vi "Book rotx_pi_2.vi"() -> ()   [LabVIEW 2013]
uses:
  <vilib>/Analysis/Matrix/Datatypes/ComplexMatrix.ctl
  <vilib>/Analysis/7linalg.llb/Real Eigenvalues and Vectors.vi
  <vilib>/robotics/Kinematics/NI_Kinematics.lvlib
  <vilib>/Analysis/NI_AALPro.lvlib
  <vilib>/picture/3D Picture Control/NI_3D Picture Control.lvlib
  <vilib>/Analysis/Matrix/NI_Matrix.lvlib
panel:
  out "rot Y * rot X":picture
  out "3D Picture 3":refnum<vi>(3d-picture)
  out "rot X * rot Y":picture
  out "3D Picture 2":refnum<vi>(3d-picture)
  out "3D Picture":refnum<vi>(3d-picture)
  out "RPY transformation":picture
  out "transformation matrix":picture
  out "Eigenvectors":T1
  out "Eigenvalues":cdb[](array[numeric])
  out "vector":dbl[](array[numeric])
  out "theta":dbl
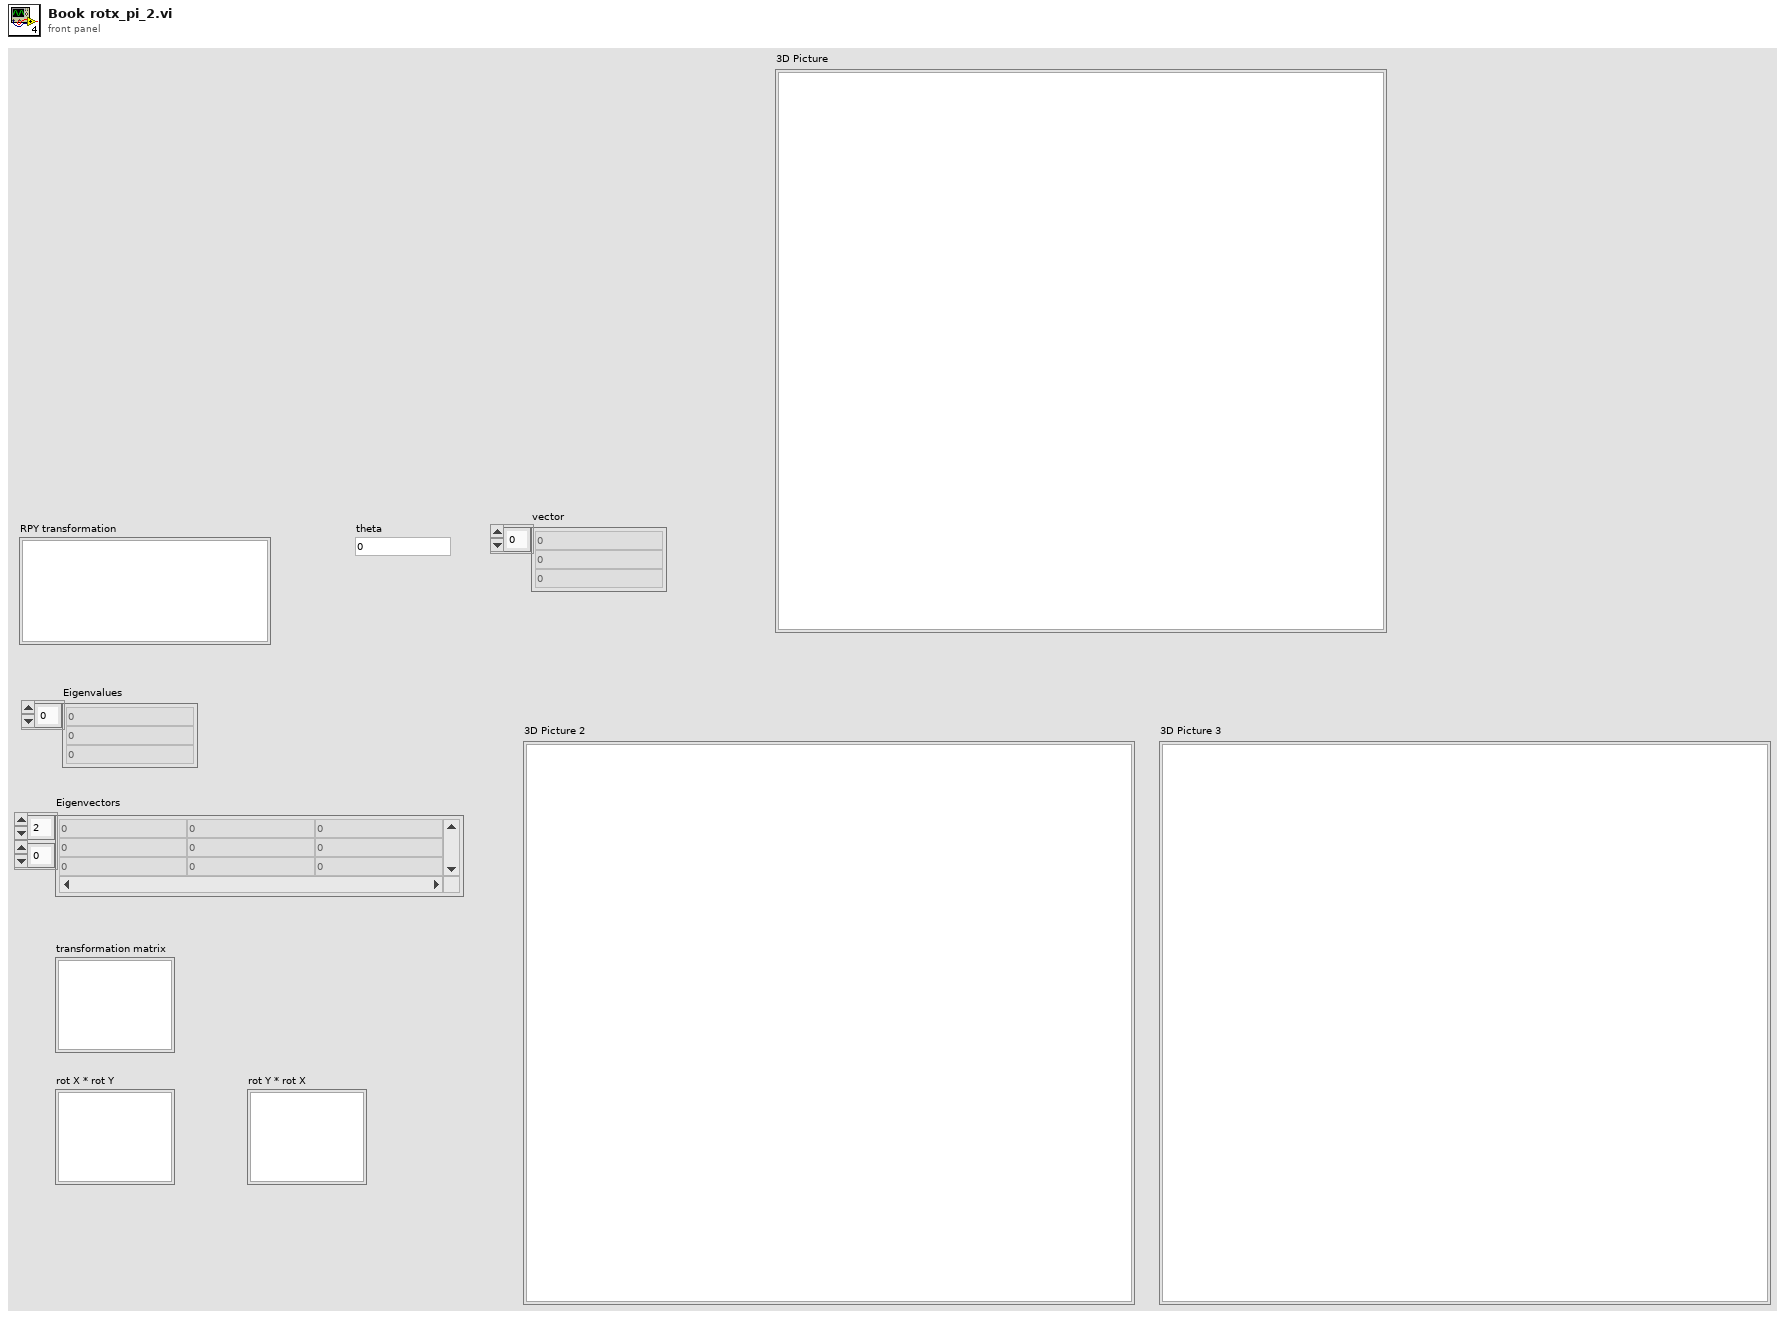
[diagram p1: front panel]
types:
  T1 = typedef "NI_Matrix.lvlib/ComplexMatrix.ctl" = cdb[][]
  T2 = typedef "NI_Matrix.lvlib/RealMatrix.ctl" = dbl[][]
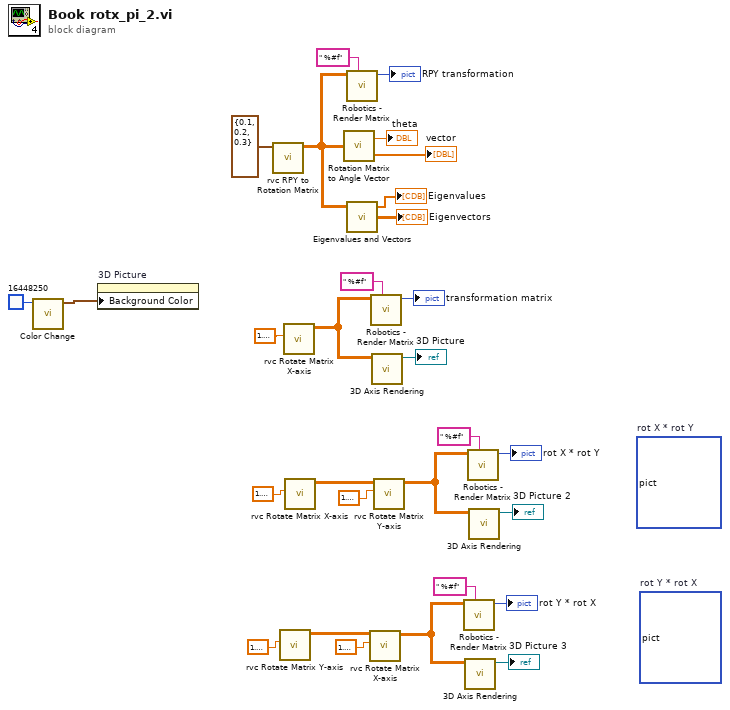
[diagram p0: block diagram]
diagram:
  (unwired) picture bytes[500]  # rot Y * rot X
  (unwired) picture bytes[500]  # rot X * rot Y
  n1 = call <vilib>:"Color Change.vi"("Color"=u32 16448250) -> ("RGBA"=w16:cluster{"R":sgl, "G":sgl, "B":sgl, "A":sgl})  [unwired: 10 in]
  n2 = property on="3D Picture" class="SceneGraphDisp (strict)"("Background Color"=w16) -> ()  [unwired: 2 in, 2 out]
  n3 = call "rvc RPY to Rotation Matrix.vi"("angles"=cluster{"roll":dbl, "pitch":dbl, "yaw":dbl} {"roll"=0.1, "pitch"=0.2, "yaw"=0.3}) -> ("rotation matrix"=w20:T2)  [unwired: 10 in]
  n4 = call "rvc Rotate Matrix Y-axis.vi"("angle"=1.5707963267948966) -> ("rotation matrix"=w2:T2)  [unwired: 10 in]
  n5 = call "rvc Rotate Matrix X-axis.vi"("angle"=1.5707963267948966) -> ("rotation matrix"=w19:T2)  [unwired: 10 in]
  n6 = call "rvc Rotate Matrix X-axis.vi"("angle"=1.5707963267948966) -> ("rotation matrix"=w13:T2)  [unwired: 10 in]
  n7 = call <vilib>:"Rotation Matrix to Angle Vector.vi"("rotation matrix"=w20) -> ("angle"=→"theta":dbl, "vector"=→"vector":dbl[])
  n8 = call "Robotics - Render Matrix.vi"("format string"=" %#f", "A"=w20) -> ("picture out"=→"RPY transformation":picture)  [unwired: 9 in]
  n9 = call-poly <vilib>:"Eigenvalues and Vectors.vi"("Input Matrix"=w20) -> ("Eigenvectors"=→"Eigenvectors":T1, "Eigenvalues"=→"Eigenvalues":cdb[])  [unwired: 2 in, 1 out]
  n10 = call "rvc Rotate Matrix X-axis.vi"("angle"=1.5707963267948966, "rotation matrix in"=w2) -> ("rotation matrix"=w1:T2)  [unwired: 9 in]
  n11 = call "Robotics - Render Matrix.vi"("format string"=" %#f", "A"=w19) -> ("picture out"=→"transformation matrix":picture)  [unwired: 9 in]
  n12 = call "3D Axis Rendering.vi"("rotation matrix"=w19) -> ("SceneNode out"=→"3D Picture":refnum<vi>)  [unwired: 9 in, 1 out]
  n13 = call "rvc Rotate Matrix Y-axis.vi"("angle"=1.5707963267948966, "rotation matrix in"=w13) -> ("rotation matrix"=w9:T2)  [unwired: 9 in]
  n14 = call "Robotics - Render Matrix.vi"("format string"=" %#f", "A"=w1) -> ("picture out"=→"rot Y * rot X":picture)  [unwired: 9 in]
  n15 = call "3D Axis Rendering.vi"("rotation matrix"=w1) -> ("SceneNode out"=→"3D Picture 3":refnum<vi>)  [unwired: 9 in, 1 out]
  n16 = call "Robotics - Render Matrix.vi"("format string"=" %#f", "A"=w9) -> ("picture out"=→"rot X * rot Y":picture)  [unwired: 9 in]
  n17 = call "3D Axis Rendering.vi"("rotation matrix"=w9) -> ("SceneNode out"=→"3D Picture 2":refnum<vi>)  [unwired: 9 in, 1 out]
